vi "Current Stamp.vi"(7 "Get/Set":enum16{"Get", "Set"}(ring), 8 "error in (no error)":errorcluster, 9 "New Stamp":string, 11 "FlexWorktable in":refnum<class "FlexWorktable.lvclass">) -> (0 "error out":errorcluster, 1 "Current Stamp":string, 3 "FlexWorktable out":refnum<class "FlexWorktable.lvclass">)   [LabVIEW 2017, in "FlexWorktable.lvclass"]
uses:
  FlexWorktable.lvclass
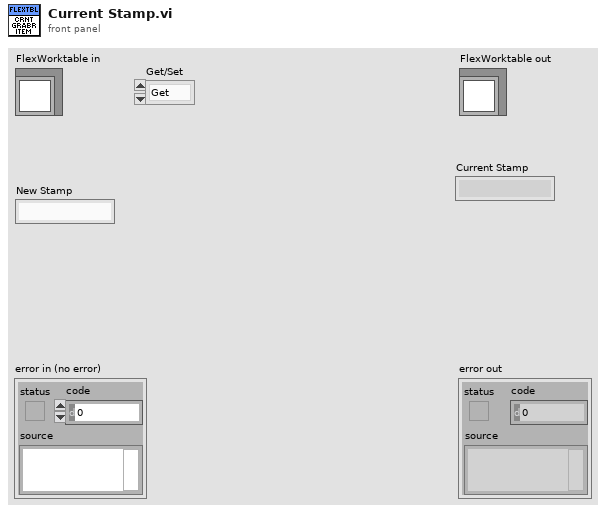
[diagram p1: front panel]
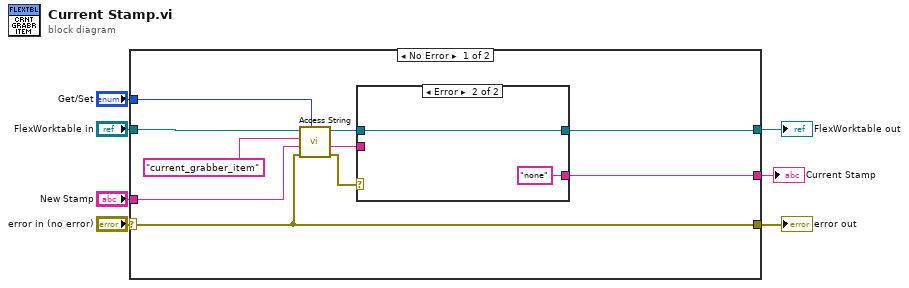
[diagram p0: block diagram]
diagram:
  n1 = case shown="No Error" "error in (no error)" {
    selector: "error in (no error)" -> [w8 w23]
    tunnel: [w8 w23] -> w6
    tunnel: [w9 w22] -> w4
    tunnel: "FlexWorktable in" -> [w17 w22]
    tunnel: "Get/Set" -> [w15 _]
    tunnel: "New Stamp" -> [w14 _]
    tunnel: [w10 _] -> w1
    frame No Error {
      n2 = call-dynamic "Access String.vi"("Get/Set"=w15, "error in (no error)"=w8, "Value in"=w14, "Key"="current_grabber_item", "FlexWorktable in"=w17) -> ("error out"=w11:errorcluster, "Value out"=w13:string, "FlexWorktable out"=w12:refnum<class "FlexWorktable.lvclass">)  [unwired: 4 in]
      n3 = case shown="Error" w11 {
        tunnel: w13 -> [w18 _]
        tunnel: w12 -> [w19 w20]
        tunnel: [w19 w20] -> w9
        tunnel: [w18 "none" ("Value out")] -> w10
        frame No Error {
        }
        frame Error {
        }
      }
    }
    frame Error {
    }
  }
  "error out" <- w6
  "FlexWorktable out" <- w4
  "Current Stamp" <- w1
